vi "Door Open Interlock Value Change.vi"(8 "error in (no error)":errorcluster, 10 "Door Open Interlock":bool, 11 "Doors Open in":refnum<class "Doors Open.lvclass">) -> (0 "error out":errorcluster, 3 "Doors Open out":refnum<class "Doors Open.lvclass">)   [LabVIEW 2020, in "Door Controller.lvlib" / "Doors Open.lvclass"]
uses:
  Doors Open.lvclass
  C:/Users/Thomas.McQuillan/Desktop/Elevator Door Control/Door Controller/Door Controller/Door Controller.lvclass
  Application/Application/Interlock Names.ctl
  Door Controller/Door Controller.lvclass
  Application/Application.lvlib
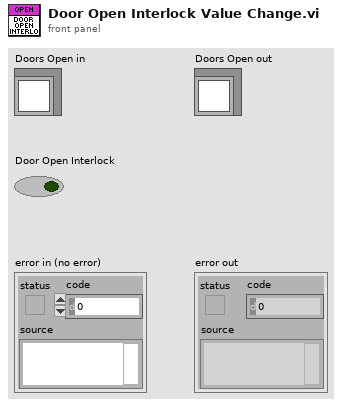
[diagram p1: front panel]
types:
  T1 = typedef "Application.lvlib/Interlock Names.ctl" = enum16{"Door Closed Interlock", "Door Open Interlock"}
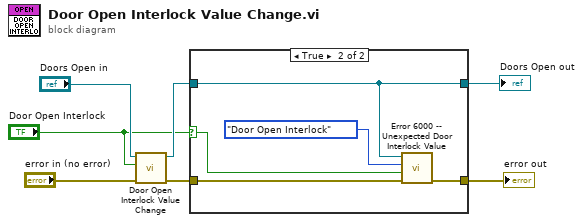
[diagram p0: block diagram]
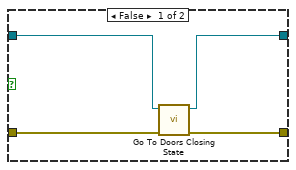
[diagram p2: hidden frame]
diagram:
  n1 = call-parent "Door Open Interlock Value Change.vi"("error in (no error)"="error in (no error)", "Door Open Interlock"="Door Open Interlock", "Door Controller in"="Doors Open in") -> ("error out"=w2:errorcluster, "Door Controller out"=w5:refnum<class "Doors Open.lvclass">)  [unwired: 7 in]
  n2 = case shown="True" "Door Open Interlock" {
    selector: "Door Open Interlock" -> [_ w14]
    tunnel: w5 -> [w11 w12]
    tunnel: [w10 w12] -> w4
    tunnel: w2 -> [w9 w15]
    tunnel: [w8 w13] -> w1
    frame False {
      n3 = call "Go To Doors Closing State.vi"("error in (no error)"=w9, "Door Controller in"=w11) -> ("error out"=w8:errorcluster, "Door Controller out"=w10:refnum<class "Doors Open.lvclass">)  [unwired: 8 in]
    }
    frame True {
      n4 = call "Error 6000 -- Unexpected Door Interlock Value.vi"("error in (no error)"=w15, "Interlock Value"=w14, "Interlock Name"=Interlock_Names."Door Open Interlock", "Door Controller"=w12) -> ("error out"=w13:errorcluster)  [unwired: 7 in]
    }
  }
  "error out" <- w1
  "Doors Open out" <- w4
